vi "CH2.vi"() -> ()   [LabVIEW 2021]
panel:
  in  "CH2":cluster{"CH2 Array":dbl[], "CH2 Message":string}
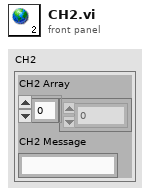
[diagram p1: front panel]
diagram:
